vi "Pre Launch Init.vi"(11 "Valve in":refnum<class "Valve.lvclass">) -> (0 "error out":errorcluster, 3 "Valve out":refnum<class "Valve.lvclass">)   [LabVIEW 2015, in "cRIO-Carbondioxide.lvlib" / "CO2-Actor.lvlib" / "Valve.lvclass"]
doc: "(<B>Filename</B>: Actor Framework.lvlib:Actor.lvclass:Pre Launch Init.vi)\n\nDefines behavior that occurs after the Launch Actor method is invoked but before the actor's Actor Core method begins running.\n\nThe Pre Launch Init method is guaranteed to finish before the Launch Actor method returns to its caller and before the actor itself receives any messages. Any references that the Pre Launch Init method obtains are guaranteed to have the same lifetime as the actor itself. Any errors that the Pre Launch Init method returns will abort the launch.\n\nBy default, this method does nothing. A descendant class may override it to define behavior."
uses:
  Valve.lvclass
  Valve.lvclass/Valve.ctl
  CO2 Actor/CO2 Actor.lvclass/CO2 Actor.ctl
  CO2 Actor/CO2 Actor.lvclass
  Interlocks/Interlock Chain/Interlock Chain.lvclass
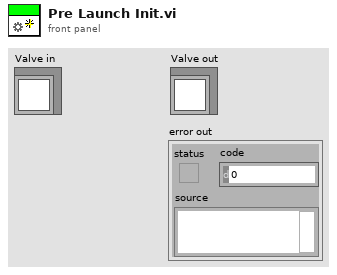
[diagram p1: front panel]
types:
  T1 = typedef "Action.ctl" = enum16{"Open", "Close", "None"}
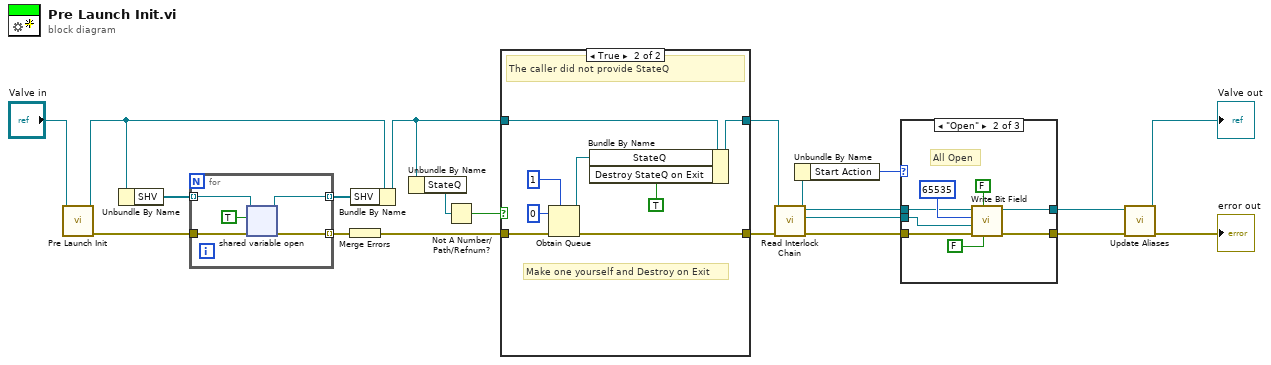
[diagram p0: block diagram]
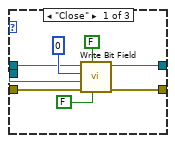
[diagram p2: hidden frame]
diagram:
  n1 = call-parent "Pre Launch Init.vi"("CO2 Actor in"="Valve in") -> ("error out"=w18:errorcluster, "CO2 Actor out"=w16:refnum<class "Valve.lvclass">)  [unwired: 9 in]
  n2 = Unbundle By Name(w16) -> ("SHV"=w19:refnum<k21>[])
  n3 = for {
    tunnel: w19 -> [w24] mode=indexing
    tunnel: w18 -> [w25]
    tunnel: [w22] -> w17 mode=indexing
    tunnel: [w23] -> w15 mode=indexing
    n4 = shared-variable-open(w24, w25, TRUE) -> (w23:refnum<k21>, w22:errorcluster)  [unwired: 1 in]
  }
  n5 = Merge Errors(w17) -> (w5:errorcluster)
  n6 = Bundle By Name(cluster=w16, "SHV"=w15) -> (w7:refnum<class "Valve.lvclass">)
  n7 = Unbundle By Name(w7) -> ("StateQ"=w8:refnum<queue>)
  n8 = Not A Number/Path/Refnum?(number/path/refnum=w8) -> (NaN/Path/Refnum?=w3:bool)
  n9 = case shown="True" w3 {
    tunnel: w7 -> [w27 w30]
    tunnel: [w27 w29] -> w6
    tunnel: w5 -> [w26 w35]
    tunnel: [w26 w34] -> w4
    frame False {
    }
    frame True {
      # "Make one yourself and Destroy on Exit"
      # "The caller did not provide StateQ"
      n10 = Obtain Queue(max queue size (-1, unlimited)=1, element data type=u16 0, error in (no error)=w35) -> (queue out=w33:refnum<queue>, error out=w34:errorcluster)  [unwired: 2 in, 1 out]
      n11 = Bundle By Name(cluster=w30, "StateQ"=w33, "Destroy StateQ on Exit"=TRUE) -> (w29:refnum<class "Valve.lvclass">)
    }
  }
  n12 = call "Read Interlock Chain.vi"("error in (no error)"=w4, "CO2 Actor in"=w6) -> ("error out"=w10:errorcluster, "Interlock Chain"=w9:refnum<class "Interlock Chain.lvclass">, "CO2 Actor out"=w2:refnum<class "Valve.lvclass">)  [unwired: 7 in]
  n13 = Unbundle By Name(w2) -> ("Start Action"=w1:T1)
  n14 = case shown="\"Open\"" w1 {
    tunnel: [w42 w50 w52] -> w14
    tunnel: [w41 w49 w53] -> w12
    tunnel: w10 -> [w40 w48 w52]
    tunnel: w9 -> [w39 w44 _]
    tunnel: w2 -> [w36 w45 w53]
    frame "Close" {
      n15 = call "Write Bit Field.vi"("IL Echo(true)"=FALSE ("Echo(true)"), "Close IL Connections (T)"=FALSE, "error in (no error)"=w40, "Interlock Chain"=w39, "Bit Field"=u16 0, "Valve in"=w36) -> ("error out"=w42:errorcluster, "Valve out"=w41:refnum<class "Valve.lvclass">)  [unwired: 3 in, 1 out]
    }
    frame "Open" {
      # "All Open"
      n16 = call "Write Bit Field.vi"("IL Echo(true)"=FALSE ("Echo(true)"), "Close IL Connections (T)"=FALSE, "error in (no error)"=w48, "Interlock Chain"=w44, "Bit Field"=u16 65535, "Valve in"=w45) -> ("error out"=w50:errorcluster, "Valve out"=w49:refnum<class "Valve.lvclass">)  [unwired: 3 in, 1 out]
    }
    frame "None" {
    }
  }
  n17 = call "Update Aliases.vi"("error in (no error)"=w14, "Valve in"=w12) -> ("error out"=→"error out":errorcluster, "Valve out"=→"Valve out":refnum<class "Valve.lvclass">)  [unwired: 8 in]
